vi "part number.vi"() -> ()   [LabVIEW 2019]
uses:
  save.ctl
panel:
  in  "partnumber":T1
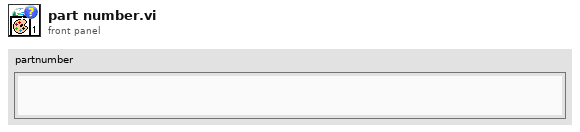
[diagram p1: front panel]
types:
  T1 = typedef "save.ctl" = string
diagram:
